vi "Z-Transform Delay Node.vi"   [LabVIEW 2017]
doc: "Stores data from one VI execution or loop iteration to the next. This node is the Feedback Node in z-transform view."
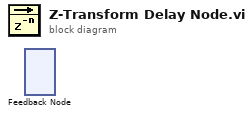
[diagram p0: block diagram]
diagram:
  n1 = feedback-in #1() -> ()  [unwired: 1 out]
  n2 = feedback #1() -> ()  [unwired: 2 in]
